vi "Decoder.vi"(8 "error in (no error)":errorcluster, 11 "StepMotor in":refnum<class "StepMotor.lvclass">) -> (0 "error out":errorcluster, 3 "StepMotor out":refnum<class "StepMotor.lvclass">)   [LabVIEW 2010, in "StepMotor.lvclass"]
doc: "Декодирование сообщения"
uses:
  StepMotor.lvclass
  StepMotor.lvclass/StepMotor.ctl
panel:
  out "SUB":bool
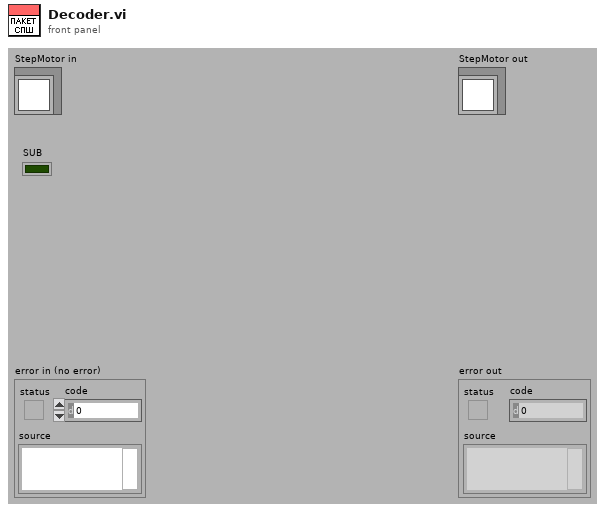
[diagram p1: front panel]
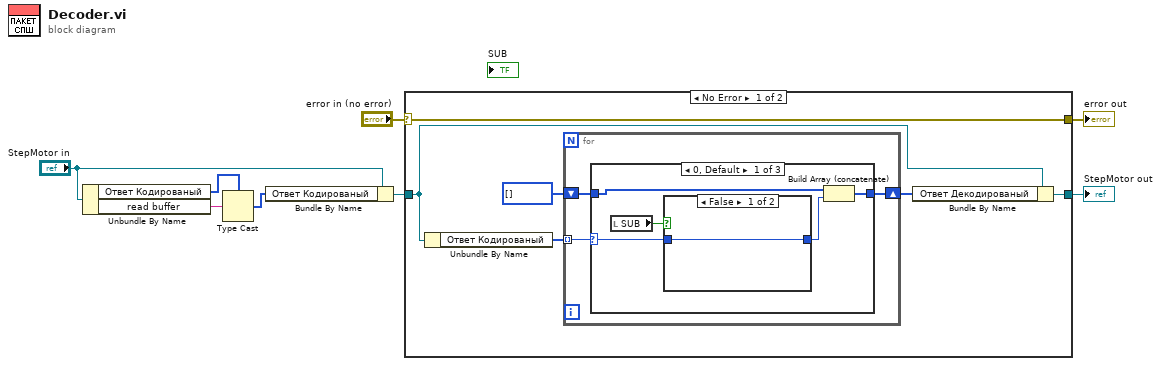
[diagram p0: block diagram]
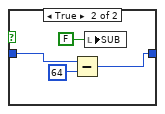
[diagram p2: hidden frame]
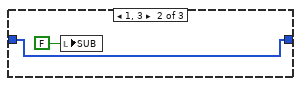
[diagram p3: hidden frame]
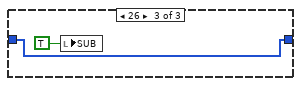
[diagram p4: hidden frame]
diagram:
  n1 = Unbundle By Name("StepMotor in") -> ("Ответ Кодированый"=w4:u8[], "read buffer"=w5:string)
  n2 = Type Cast(type=w4, x=w5) -> (*(type *) &x=w2:u8[])
  n3 = Bundle By Name(cluster="StepMotor in", "Ответ Кодированый"=w2) -> (w1:refnum<class "StepMotor.lvclass">)
  n4 = case shown="No Error" "error in (no error)" {
    selector: "error in (no error)" -> [w14 w33]
    tunnel: [w14 w33] -> w7
    tunnel: [w10 w32] -> w6
    tunnel: w1 -> [w9 w32]
    frame No Error {
      n5 = Unbundle By Name(w9) -> ("Ответ Кодированый"=w12:u8[])
      n6 = for {
        tunnel: w12 -> [w17] mode=indexing
        shift-right: [w15] -> w11
        shift-left: u8[] [] ("appended array") -> [w16]
        n7 = case shown="0, Default" w17 {
          selector: w17 -> [w19 _ _]
          tunnel: w16 -> [w22 w29 w30]
          tunnel: [w21 w29 w30] -> w15
          frame 0, Default {
            n8 = local read "SUB"() -> (w20:bool)
            n9 = case shown="False" w20 {
              tunnel: [w23 w25] -> w18
              tunnel: w19 -> [w23 w26]
              frame False {
              }
              frame True {
                n10 = Subtract(x=w26, y=u8 64 ("Numeric")) -> (x-y=w25:u8)
                n11 = local write "SUB"(FALSE ("SUB")) -> ()
              }
            }
            n12 = Build Array (concatenate)(w22, w18) -> (w21:u8[])
          }
          frame 1, 3 {
            n13 = local write "SUB"(FALSE ("SAB")) -> ()
          }
          frame 26 {
            n14 = local write "SUB"(TRUE ("SAB")) -> ()
          }
        }
      }
      n15 = Bundle By Name(cluster=w9, "Ответ Декодированый"=w11) -> (w10:refnum<class "StepMotor.lvclass">)
    }
    frame Error {
    }
  }
  "error out" <- w7
  "StepMotor out" <- w6
